vi "ex_2.vi"() -> ()   [LabVIEW 2020]
panel:
  out "Time elapsed":string
  in  "stop button":bool
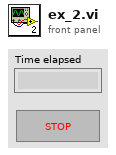
[diagram p1: front panel]
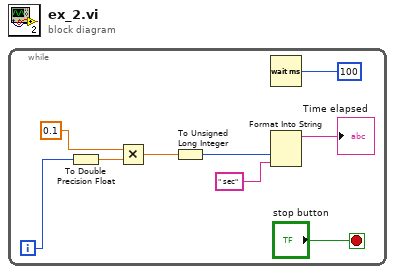
[diagram p0: block diagram]
diagram:
  n1 = while {
    i -> [w5]
    stop <- "stop button" stop-if-true
    n2 = To Double Precision Float(number=w5) -> (double precision float=w4:dbl)
    n3 = Multiply(x=0.1, y=w4) -> (x*y=w6:dbl)
    n4 = To Unsigned Long Integer(number=w6) -> (unsigned 32bit integer=w3:u32)
    n5 = Wait (ms)(milliseconds to wait=u32 100) -> ()  [unwired: 1 out]
    n6 = Format Into String(w3, " sec") -> (resulting string=→"Time elapsed":string)  [unwired: 3 in, 1 out]
  }
